vi "subDAQ_SetLED.vi"(6 "DAQ ports":T2={"Lasers DO lines"=["Dev2/port0/line0", "Dev2/port0/line1", "Dev2/port0/line2", "Dev2/port0/line3", "Dev2/port0/line4", "Dev2/port0/line5"], "Lasers AO lines"=["Dev2/ao0", "Dev2/ao1", "Dev2/ao2", "Dev2/ao3", "Dev2/ao4", "Dev2/ao5"], "Patch AO line"="Dev1/ao1", "Patch AI lines 1"={"Patch scaled output"="Dev1/ai8", "Patch 10 V_m "="Dev1/ai0"}, "Camera timing DI"="Dev1/port0/line8", "Dev1 timing DO "="Dev1/port0/line9", "Dev1 trigger source"="/Dev1/PFI0", "Dev2 trigger source"="/Dev2/PFI0", "LED line"="Dev1/port0/line0", "Global Shutter line"="Dev2/port0/line6", "Patch AI lines 2"={"Cell capacitance"="Dev1/ai1", "Mode"="Dev1/ai2", "Frequency"="Dev1/ai3", "Gain"="Dev1/ai4"}}, 7 "Light control (All Off)":T1={"Filter Set"=4, "Lasers DO"=[FALSE, FALSE, FALSE, FALSE, FALSE, FALSE], "Lasers AO (V)"=[0.0, 0.0, 0.0, 0.0, 0.0, 0.0], "LED"=FALSE, "Global"=FALSE} {"Lasers AO (V)" min=0.0 max=5.0 step=0.01 scale=0.0..5.0 scale format="%#1.2f"; "Filter Set" items=["R-QuasAr", "R-Cy5", "R-mCherry", "R-mOrange", "R-GFP", "R-CFP/DAPI", "R-BFP", "R-LED", "SDC-Cy5", "SDC-mCherry", "SDC-mO2", "SDC-GFP", "SDC-CFP/DAPI", "SDC-BFP", "SDC-LED"]}, 8 "Error in (no error)":errorcluster) -> (0 "Error out":errorcluster)   [LabVIEW 2015]
panel:
  # "Red"
  # "637"
  # "561"
  # "488"
  # "405"
  # "532"
  # "637"
  # "561"
  # "532"
  # "488"
  # "405"
  # "Red"
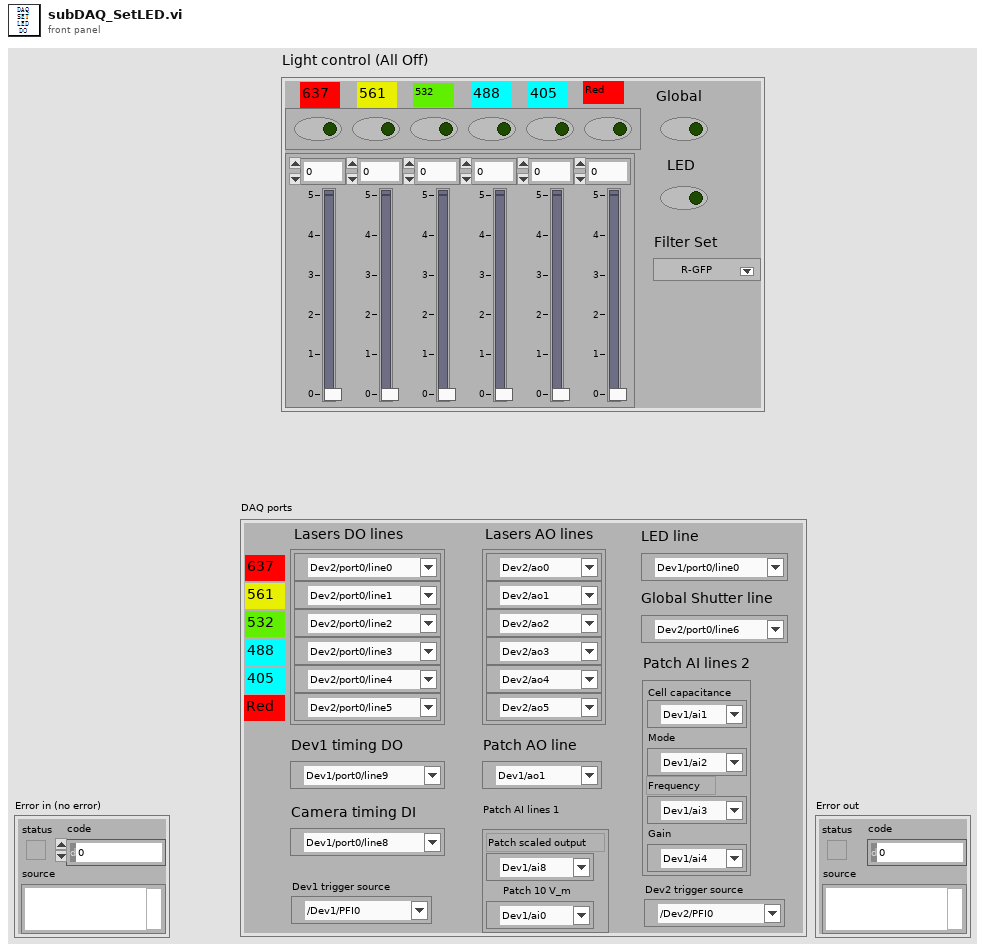
[diagram p1: front panel]
types:
  T1 = cluster{"Filter Set":i32, "Lasers DO":bool[], "Lasers AO (V)":dbl[], "LED":bool, "Global":bool}
  T2 = cluster{"Lasers DO lines":tag[], "Lasers AO lines":tag[], "Patch AO line":tag, "Patch AI lines 1":cluster{"Patch scaled output":tag, "Patch 10 V_m ":tag}, "Camera timing DI":tag, "Dev1 timing DO ":tag, "Dev1 trigger source":tag, "Dev2 trigger source":tag, "LED line":tag, "Global Shutter line":tag, "Patch AI lines 2":cluster{"Cell capacitance":tag, "Mode":tag, "Frequency":tag, "Gain":tag}}
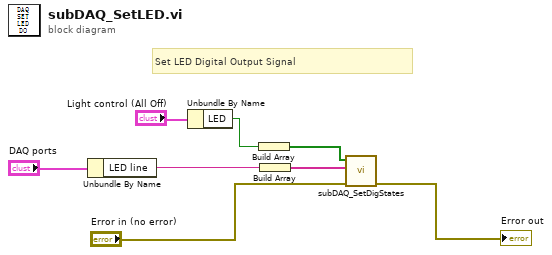
[diagram p0: block diagram]
diagram:
  # "Set LED Digital Output Signal"
  n1 = Unbundle By Name("DAQ ports") -> ("LED line"=w7:tag)
  n2 = Unbundle By Name("Light control (All Off)") -> ("LED"=w1:bool)
  n3 = Build Array(w1) -> (w5:bool[])
  n4 = Build Array(w7) -> (w6:tag[])
  n5 = call "subDAQ_SetDigStates.vi"("Error in (no error)"="Error in (no error)", "Digital line array"=w6, "Digital States (Value) array"=w5) -> ("Error out"=→"Error out":errorcluster)  [unwired: 8 in]
